vi "Check output file.vi"() -> ()   [LabVIEW 2016]
panel:
  out "size(s)":i32
  in  "Output channel name":string="Output"
  out "Array sizes":i32[](array[numeric])=[2502, 2502, 2502, 2502, 2502]
  out "Waveform Graph":dbl[][](graph)
  out "Array - Numeric":dbl[][](array[numeric])
  in  "channel name(s) in":string="Frequency"
  in  "Array":path[](array[path])=[path "C:/Data/March_2017/030717/ru001_030717.tdms", path "C:/Data/March_2017/030717/ru002_030717.tdms", path "C:/Data/March_2017/030717/ru003_030717.tdms", path "C:/Data/March_2017/030717/ru004_030717.tdms", path "C:/Data/March_2017/030717/ru005_030717.tdms"]
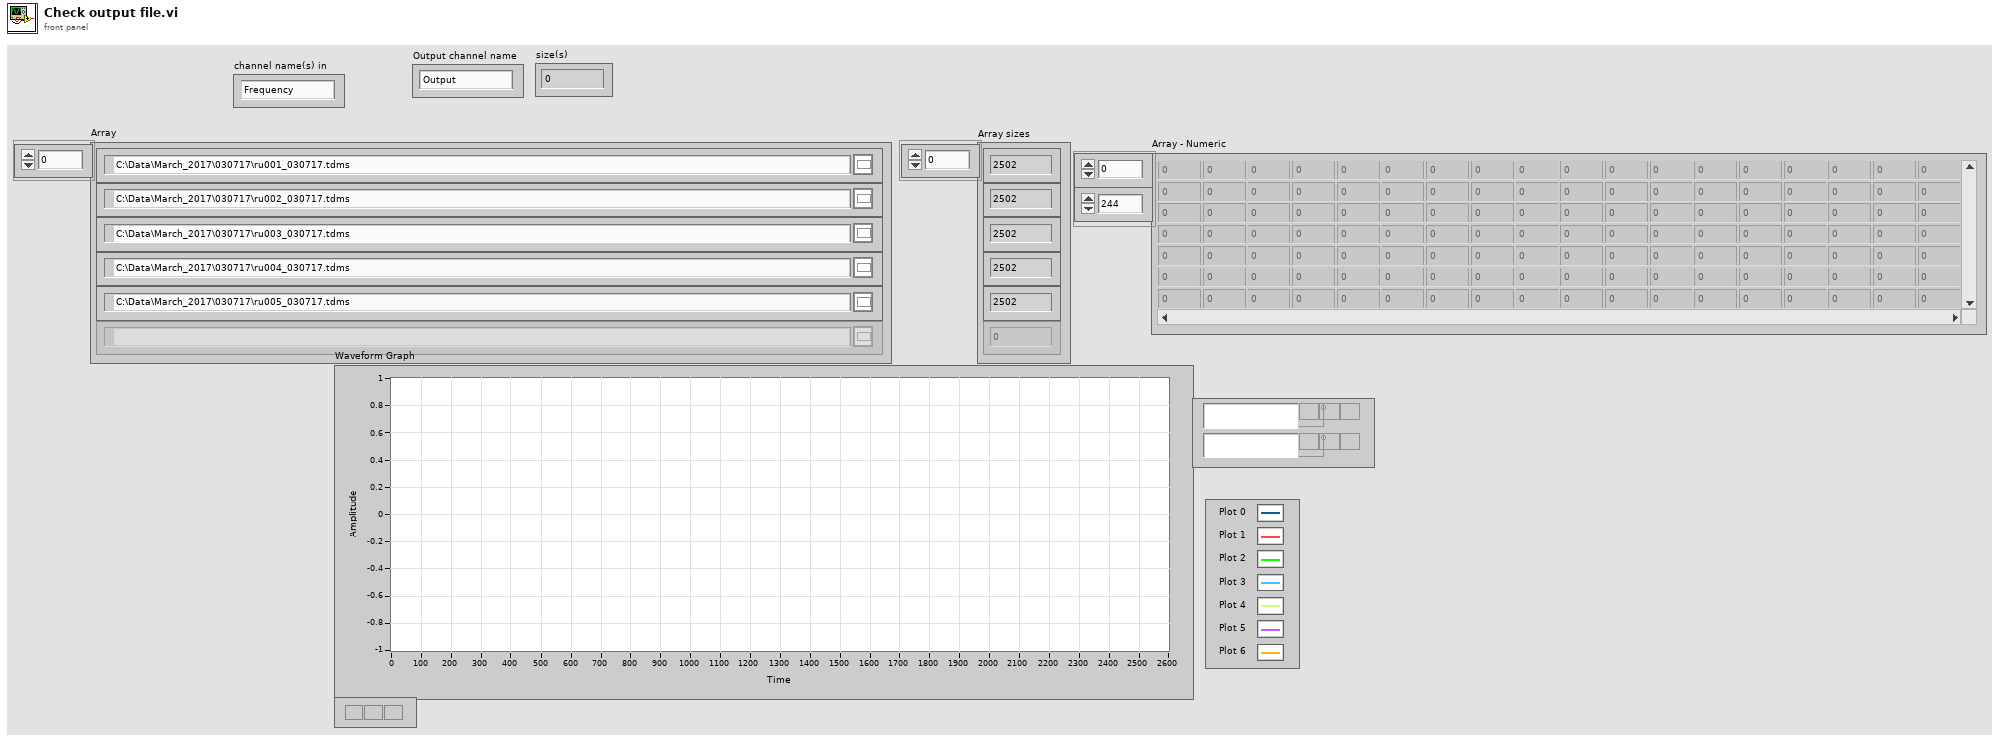
[diagram p1: front panel]
types:
  T1 = enum16{"open", "open or create", "create or replace", "create", "open (read-only)"}
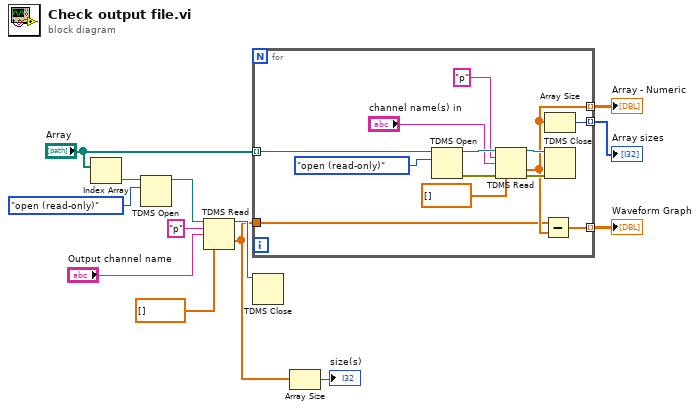
[diagram p0: block diagram]
diagram:
  n1 = Index Array(array="Array") -> (element=w3:path)  [unwired: 1 in]
  n2 = TDMS Open(10:T1."open (read-only)" ("operation (0:open)"), 11:w3) -> (3:w7:refnum<k34>)  [unwired: 5 in, 1 out]
  n3 = TDMS Read(0:w7, 5:"p" ("group name in"), 7:"Output channel name", 12:dbl[] []) -> (4:w9:refnum<k34>, 10:w2:dbl[])  [unwired: 4 in, 4 out]
  n4 = for {
    tunnel: "Array" -> [w26] mode=indexing
    tunnel: [w16] -> w13 mode=indexing
    tunnel: [w17] -> w12 mode=indexing
    tunnel: [w15] -> w11 mode=indexing
    tunnel: w2 -> [w14]
    n5 = TDMS Open(10:T1."open (read-only)" ("operation (0:open)"), 11:w26) -> (0:w23:errorcluster, 3:w24:refnum<k34>)  [unwired: 5 in]
    n6 = TDMS Read(0:w24, 5:"p" ("group name in"), 7:"channel name(s) in", 11:w23, 12:dbl[] []) -> (4:w19:refnum<k34>, 10:w16:dbl[], 15:w18:errorcluster)  [unwired: 3 in, 3 out]
    n7 = Subtract(x=w14, y=w16) -> (x-y=w17:dbl[])
    n8 = Array Size(array=w16) -> (size(s)=w15:i32)
    n9 = TDMS Close(8:w18, 11:w19) -> ()  [unwired: 2 out]
  }
  "Array - Numeric" <- w13
  "Waveform Graph" <- w12
  "Array sizes" <- w11
  n10 = TDMS Close(11:w9) -> ()  [unwired: 1 in, 2 out]
  n11 = Array Size(array=w2) -> (size(s)=→"size(s)":i32)
